vi "S4GUI.vi"() -> ()   [LabVIEW 2018] (continued)
            n2475 = call "Read WPROT.vi"("error in (no error)"=w5896, "Instrument in"=w5899) -> ("error out"=w5895:errorcluster, "Opt_Selector.lvclass"=w5897:refnum<class "Opt_Selector.lvclass">, "Instrument out"=w5898:refnum<class "Instrument.lvclass">)  [unwired: 7 in]
            n2476 = call-dynamic "Read sequencia_ant.vi"("error in (no error)"=w5895, "Opt_Selector in"=w5897) -> ("error out"=w5891:errorcluster, "sequencia_ant"=w5890:u16, "Opt_Selector out"=w5892:refnum<class "Opt_Selector.lvclass">)  [unwired: 7 in]
            n2477 = call-dynamic "Write sequencia.vi"("error in (no error)"=w5891, "sequencia"=w5890, "Opt_Selector in"=w5892) -> ("error out"=w5878:errorcluster, "Opt_Selector out"=w5881:refnum<class "Opt_Selector.lvclass">)  [unwired: 7 in]
            n2478 = call-dynamic "Read State Machine.vi"("error in (no error)"=w5878, "Device in"=w5881) -> ("error out"=w5883:errorcluster, "State Machine.lvclass"=w5886:refnum<class "State Machine.lvclass">, "Device out"=w5880:refnum<class "Opt_Selector.lvclass">)  [unwired: 7 in]
            n2479 = call "Next State.vi"("error in (no error)"=w5883, "New_State"=10, "State Machine in"=w5886) -> ("error out"=w5882:errorcluster, "State Machine out"=w5885:refnum<class "State Machine.lvclass">)  [unwired: 7 in]
            n2480 = call-dynamic "Write State Machine.vi"("error in (no error)"=w5882, "State Machine.lvclass"=w5885, "Device in"=w5880) -> ("error out"=w5877:errorcluster, "Device out"=w5879:refnum<class "Opt_Selector.lvclass">)  [unwired: 7 in]
            n2481 = call "Write WPROT.vi"("error in (no error)"=w5877, "Opt_Selector.lvclass"=w5879, "Instrument in"=w5898) -> ("error out"=w5894:errorcluster, "Instrument out"=w5893:refnum<class "Instrument.lvclass">)  [unwired: 7 in]
            n2482 = call "Write Instrument.lvclass.vi"("error in (no error)"=w5894, "Instrument.lvclass"=w5893, "S4ACS_GUI in"=w5900) -> ("error out"=w5888:errorcluster, "S4ACS_GUI out"=w5876:refnum<class "S4GUI.lvclass">)  [unwired: 7 in]
          }
          frame Enabled {
            w5931 = FALSE ("Wait Until Done")
            n2483 = call <vilib>:"Application Directory.vi"() -> ("Application Directory"=w5934:path)
            n2484 = Build Path(base path=w5934, name or relative path="MsgStop1.vi") -> (appended path=w5935:path)
            n2485 = Open VI Reference(vi path=w5935, error in (no error)=w5929) -> (vi reference=w5933:refnum<vi>, error out=w5932:errorcluster)  [unwired: 4 in]
            n2486 = invoke class="VI" method="Run VI"(reference=w5933, error in=w5932, "Wait until done"=w5931, "Auto Dispose Ref"=w5931) -> (error out=w5928:errorcluster)  [unwired: 1 in, 4 out]
          }
        }
      }
      event "Stop ch2": Value Change {
        n2487 = event-data() -> ()  [unwired: 1 in, 6 out]
        n2488 = disable-structure shown="Enabled" {
          disable-tunnel: w5940 -> [w5973 w5993]
          disable-tunnel: w5939 -> [w5971 w5995]
          disable-tunnel: [w5953 w5994] -> w5938
          disable-tunnel: [w5941 w5993] -> w5937
          frame Disabled {
            # "Para movimento \nda lamina retardadora"
            # "Restaura a última sequência de lâminas"
            n2489 = call "Read AcquisitionB.vi"("error in (no error)"=w5971, "S4ACS_GUI in"=w5973) -> ("error out"=w5975:errorcluster, "Acquisition.lvclass"=w5974:refnum<class "Acquisition.lvclass">, "S4ACS_GUI out"=w5972:refnum<class "S4GUI.lvclass">)  [unwired: 7 in]
            n2490 = disable-structure shown="Enabled" {
              disable-tunnel: w5975 -> [w5980 w5991]
              disable-tunnel: w5974 -> [w5979 w5992]
              disable-tunnel: [w5977 w5992] -> w5969
              disable-tunnel: [w5976 w5991] -> w5968
              frame Disabled {
                # "Só precisa enviar comando STOP quando\no controle dos ciclos for feito pelo ACS."
                n2491 = call-dynamic "Read Channel.vi"("error in (no error)"=w5980, "Acquisition in"=w5979) -> ("error out"=w5982:errorcluster, "Channel.lvclass"=w5981:refnum<class "Channel.lvclass">, "Acquisition out"=w5988:refnum<class "Acquisition.lvclass">)  [unwired: 7 in]
                n2492 = call-dynamic "Read State Machine.vi"("error in (no error)"=w5982, "Device in"=w5981) -> ("error out"=w5984:errorcluster, "State Machine.lvclass"=w5983:refnum<class "State Machine.lvclass">, "Device out"=w5986:refnum<class "Channel.lvclass">)  [unwired: 7 in]
                n2493 = call "Next State.vi"("error in (no error)"=w5984, "New_State"=u32 70, "State Machine in"=w5983) -> ("error out"=w5987:errorcluster, "State Machine out"=w5985:refnum<class "State Machine.lvclass">)  [unwired: 7 in]
                n2494 = call-dynamic "Write State Machine.vi"("error in (no error)"=w5987, "State Machine.lvclass"=w5985, "Device in"=w5986) -> ("error out"=w5989:errorcluster, "Device out"=w5990:refnum<class "Channel.lvclass">)  [unwired: 7 in]
                n2495 = call-dynamic "Write Channel.vi"("error in (no error)"=w5989, "Channel.lvclass"=w5990, "Acquisition in"=w5988) -> ("error out"=w5976:errorcluster, "Acquisition out"=w5977:refnum<class "Acquisition.lvclass">)  [unwired: 7 in]
              }
              frame Enabled {
                # "Não precisa enviar comando STOP para o ACS\nenquanto o controle dos ciclos for feito pela GUI."
              }
            }
            n2496 = call-dynamic "Write Acq_state.vi"("error in (no error)"=w5968, "Acq_state"=u32 0, "Acquisition in"=w5969) -> ("error out"=w5967:errorcluster, "Acquisition out"=w5966:refnum<class "Acquisition.lvclass">)  [unwired: 7 in]
            n2497 = call "Write AcquisitionB.vi"("error in (no error)"=w5967, "Acquisition.lvclass"=w5966, "S4ACS_GUI in"=w5972) -> ("error out"=w5954:errorcluster, "S4ACS_GUI out"=w5952:refnum<class "S4GUI.lvclass">)  [unwired: 7 in]
            n2498 = call "Read Instrument.lvclass.vi"("error in (no error)"=w5954, "S4ACS_GUI in"=w5952) -> ("error out"=w5961:errorcluster, "Instrument.lvclass"=w5964:refnum<class "Instrument.lvclass">, "S4ACS_GUI out"=w5965:refnum<class "S4GUI.lvclass">)  [unwired: 7 in]
            n2499 = call "Read WPROT.vi"("error in (no error)"=w5961, "Instrument in"=w5964) -> ("error out"=w5960:errorcluster, "Opt_Selector.lvclass"=w5962:refnum<class "Opt_Selector.lvclass">, "Instrument out"=w5963:refnum<class "Instrument.lvclass">)  [unwired: 7 in]
            n2500 = call-dynamic "Read sequencia_ant.vi"("error in (no error)"=w5960, "Opt_Selector in"=w5962) -> ("error out"=w5956:errorcluster, "sequencia_ant"=w5955:u16, "Opt_Selector out"=w5957:refnum<class "Opt_Selector.lvclass">)  [unwired: 7 in]
            n2501 = call-dynamic "Write sequencia.vi"("error in (no error)"=w5956, "sequencia"=w5955, "Opt_Selector in"=w5957) -> ("error out"=w5943:errorcluster, "Opt_Selector out"=w5946:refnum<class "Opt_Selector.lvclass">)  [unwired: 7 in]
            n2502 = call-dynamic "Read State Machine.vi"("error in (no error)"=w5943, "Device in"=w5946) -> ("error out"=w5948:errorcluster, "State Machine.lvclass"=w5951:refnum<class "State Machine.lvclass">, "Device out"=w5945:refnum<class "Opt_Selector.lvclass">)  [unwired: 7 in]
            n2503 = call "Next State.vi"("error in (no error)"=w5948, "New_State"=10, "State Machine in"=w5951) -> ("error out"=w5947:errorcluster, "State Machine out"=w5950:refnum<class "State Machine.lvclass">)  [unwired: 7 in]
            n2504 = call-dynamic "Write State Machine.vi"("error in (no error)"=w5947, "State Machine.lvclass"=w5950, "Device in"=w5945) -> ("error out"=w5942:errorcluster, "Device out"=w5944:refnum<class "Opt_Selector.lvclass">)  [unwired: 7 in]
            n2505 = call "Write WPROT.vi"("error in (no error)"=w5942, "Opt_Selector.lvclass"=w5944, "Instrument in"=w5963) -> ("error out"=w5959:errorcluster, "Instrument out"=w5958:refnum<class "Instrument.lvclass">)  [unwired: 7 in]
            n2506 = call "Write Instrument.lvclass.vi"("error in (no error)"=w5959, "Instrument.lvclass"=w5958, "S4ACS_GUI in"=w5965) -> ("error out"=w5953:errorcluster, "S4ACS_GUI out"=w5941:refnum<class "S4GUI.lvclass">)  [unwired: 7 in]
          }
          frame Enabled {
            w5997 = FALSE ("Wait Until Done")
            n2507 = call <vilib>:"Application Directory.vi"() -> ("Application Directory"=w6000:path)
            n2508 = Build Path(base path=w6000, name or relative path="MsgStop2.vi") -> (appended path=w6001:path)
            n2509 = Open VI Reference(vi path=w6001, error in (no error)=w5995) -> (vi reference=w5999:refnum<vi>, error out=w5998:errorcluster)  [unwired: 4 in]
            n2510 = invoke class="VI" method="Run VI"(reference=w5999, error in=w5998, "Wait until done"=w5997, "Auto Dispose Ref"=w5997) -> (error out=w5994:errorcluster)  [unwired: 1 in, 4 out]
          }
        }
      }
      event "Stop ch3": Value Change {
        n2511 = event-data() -> ()  [unwired: 1 in, 6 out]
        n2512 = disable-structure shown="Enabled" {
          disable-tunnel: w6005 -> [w6038 w6058]
          disable-tunnel: w6004 -> [w6036 w6060]
          disable-tunnel: [w6018 w6059] -> w6003
          disable-tunnel: [w6006 w6058] -> w6002
          frame Disabled {
            # "Para movimento \nda lamina retardadora"
            # "Restaura a última sequência de lâminas"
            n2513 = call-dynamic "Read AcquisitionC.vi"("error in (no error)"=w6036, "S4ACS_GUI in"=w6038) -> ("error out"=w6040:errorcluster, "Acquisition.lvclass"=w6039:refnum<class "Acquisition.lvclass">, "S4ACS_GUI out"=w6037:refnum<class "S4GUI.lvclass">)  [unwired: 7 in]
            n2514 = disable-structure shown="Enabled" {
              disable-tunnel: w6040 -> [w6045 w6056]
              disable-tunnel: w6039 -> [w6044 w6057]
              disable-tunnel: [w6042 w6057] -> w6034
              disable-tunnel: [w6041 w6056] -> w6033
              frame Disabled {
                # "Só precisa enviar comando STOP quando\no controle dos ciclos for feito pelo ACS."
                n2515 = call-dynamic "Read Channel.vi"("error in (no error)"=w6045, "Acquisition in"=w6044) -> ("error out"=w6047:errorcluster, "Channel.lvclass"=w6046:refnum<class "Channel.lvclass">, "Acquisition out"=w6053:refnum<class "Acquisition.lvclass">)  [unwired: 7 in]
                n2516 = call-dynamic "Read State Machine.vi"("error in (no error)"=w6047, "Device in"=w6046) -> ("error out"=w6049:errorcluster, "State Machine.lvclass"=w6048:refnum<class "State Machine.lvclass">, "Device out"=w6051:refnum<class "Channel.lvclass">)  [unwired: 7 in]
                n2517 = call "Next State.vi"("error in (no error)"=w6049, "New_State"=u32 70, "State Machine in"=w6048) -> ("error out"=w6052:errorcluster, "State Machine out"=w6050:refnum<class "State Machine.lvclass">)  [unwired: 7 in]
                n2518 = call-dynamic "Write State Machine.vi"("error in (no error)"=w6052, "State Machine.lvclass"=w6050, "Device in"=w6051) -> ("error out"=w6054:errorcluster, "Device out"=w6055:refnum<class "Channel.lvclass">)  [unwired: 7 in]
                n2519 = call-dynamic "Write Channel.vi"("error in (no error)"=w6054, "Channel.lvclass"=w6055, "Acquisition in"=w6053) -> ("error out"=w6041:errorcluster, "Acquisition out"=w6042:refnum<class "Acquisition.lvclass">)  [unwired: 7 in]
              }
              frame Enabled {
                # "Não precisa enviar comando STOP para o ACS\nenquanto o controle dos ciclos for feito pela GUI."
              }
            }
            n2520 = call-dynamic "Write Acq_state.vi"("error in (no error)"=w6033, "Acq_state"=u32 0, "Acquisition in"=w6034) -> ("error out"=w6032:errorcluster, "Acquisition out"=w6031:refnum<class "Acquisition.lvclass">)  [unwired: 7 in]
            n2521 = call-dynamic "Write AcquisitionC.vi"("error in (no error)"=w6032, "Acquisition.lvclass"=w6031, "S4ACS_GUI in"=w6037) -> ("error out"=w6019:errorcluster, "S4ACS_GUI out"=w6017:refnum<class "S4GUI.lvclass">)  [unwired: 7 in]
            n2522 = call "Read Instrument.lvclass.vi"("error in (no error)"=w6019, "S4ACS_GUI in"=w6017) -> ("error out"=w6026:errorcluster, "Instrument.lvclass"=w6029:refnum<class "Instrument.lvclass">, "S4ACS_GUI out"=w6030:refnum<class "S4GUI.lvclass">)  [unwired: 7 in]
            n2523 = call "Read WPROT.vi"("error in (no error)"=w6026, "Instrument in"=w6029) -> ("error out"=w6025:errorcluster, "Opt_Selector.lvclass"=w6027:refnum<class "Opt_Selector.lvclass">, "Instrument out"=w6028:refnum<class "Instrument.lvclass">)  [unwired: 7 in]
            n2524 = call-dynamic "Read sequencia_ant.vi"("error in (no error)"=w6025, "Opt_Selector in"=w6027) -> ("error out"=w6021:errorcluster, "sequencia_ant"=w6020:u16, "Opt_Selector out"=w6022:refnum<class "Opt_Selector.lvclass">)  [unwired: 7 in]
            n2525 = call-dynamic "Write sequencia.vi"("error in (no error)"=w6021, "sequencia"=w6020, "Opt_Selector in"=w6022) -> ("error out"=w6008:errorcluster, "Opt_Selector out"=w6011:refnum<class "Opt_Selector.lvclass">)  [unwired: 7 in]
            n2526 = call-dynamic "Read State Machine.vi"("error in (no error)"=w6008, "Device in"=w6011) -> ("error out"=w6013:errorcluster, "State Machine.lvclass"=w6016:refnum<class "State Machine.lvclass">, "Device out"=w6010:refnum<class "Opt_Selector.lvclass">)  [unwired: 7 in]
            n2527 = call "Next State.vi"("error in (no error)"=w6013, "New_State"=10, "State Machine in"=w6016) -> ("error out"=w6012:errorcluster, "State Machine out"=w6015:refnum<class "State Machine.lvclass">)  [unwired: 7 in]
            n2528 = call-dynamic "Write State Machine.vi"("error in (no error)"=w6012, "State Machine.lvclass"=w6015, "Device in"=w6010) -> ("error out"=w6007:errorcluster, "Device out"=w6009:refnum<class "Opt_Selector.lvclass">)  [unwired: 7 in]
            n2529 = call "Write WPROT.vi"("error in (no error)"=w6007, "Opt_Selector.lvclass"=w6009, "Instrument in"=w6028) -> ("error out"=w6024:errorcluster, "Instrument out"=w6023:refnum<class "Instrument.lvclass">)  [unwired: 7 in]
            n2530 = call "Write Instrument.lvclass.vi"("error in (no error)"=w6024, "Instrument.lvclass"=w6023, "S4ACS_GUI in"=w6030) -> ("error out"=w6018:errorcluster, "S4ACS_GUI out"=w6006:refnum<class "S4GUI.lvclass">)  [unwired: 7 in]
          }
          frame Enabled {
            w6062 = FALSE ("Wait Until Done")
            n2531 = call <vilib>:"Application Directory.vi"() -> ("Application Directory"=w6065:path)
            n2532 = Build Path(base path=w6065, name or relative path="MsgStop3.vi") -> (appended path=w6066:path)
            n2533 = Open VI Reference(vi path=w6066, error in (no error)=w6060) -> (vi reference=w6064:refnum<vi>, error out=w6063:errorcluster)  [unwired: 4 in]
            n2534 = invoke class="VI" method="Run VI"(reference=w6064, error in=w6063, "Wait until done"=w6062, "Auto Dispose Ref"=w6062) -> (error out=w6059:errorcluster)  [unwired: 1 in, 4 out]
          }
        }
      }
      event "Stop ch4": Value Change {
        n2535 = event-data() -> ()  [unwired: 1 in, 6 out]
        n2536 = disable-structure shown="Enabled" {
          disable-tunnel: w6070 -> [w6103 w6123]
          disable-tunnel: w6069 -> [w6101 w6125]
          disable-tunnel: [w6083 w6124] -> w6068
          disable-tunnel: [w6071 w6123] -> w6067
          frame Disabled {
            # "Para movimento \nda lamina retardadora"
            # "Restaura a última sequência de lâminas"
            n2537 = call-dynamic "Read AcquisitionD.vi"("error in (no error)"=w6101, "S4ACS_GUI in"=w6103) -> ("error out"=w6105:errorcluster, "Acquisition.lvclass"=w6104:refnum<class "Acquisition.lvclass">, "S4ACS_GUI out"=w6102:refnum<class "S4GUI.lvclass">)  [unwired: 7 in]
            n2538 = disable-structure shown="Enabled" {
              disable-tunnel: w6105 -> [w6110 w6121]
              disable-tunnel: w6104 -> [w6109 w6122]
              disable-tunnel: [w6107 w6122] -> w6099
              disable-tunnel: [w6106 w6121] -> w6098
              frame Disabled {
                # "Só precisa enviar comando STOP quando\no controle dos ciclos for feito pelo ACS."
                n2539 = call-dynamic "Read Channel.vi"("error in (no error)"=w6110, "Acquisition in"=w6109) -> ("error out"=w6112:errorcluster, "Channel.lvclass"=w6111:refnum<class "Channel.lvclass">, "Acquisition out"=w6118:refnum<class "Acquisition.lvclass">)  [unwired: 7 in]
                n2540 = call-dynamic "Read State Machine.vi"("error in (no error)"=w6112, "Device in"=w6111) -> ("error out"=w6114:errorcluster, "State Machine.lvclass"=w6113:refnum<class "State Machine.lvclass">, "Device out"=w6116:refnum<class "Channel.lvclass">)  [unwired: 7 in]
                n2541 = call "Next State.vi"("error in (no error)"=w6114, "New_State"=u32 70, "State Machine in"=w6113) -> ("error out"=w6117:errorcluster, "State Machine out"=w6115:refnum<class "State Machine.lvclass">)  [unwired: 7 in]
                n2542 = call-dynamic "Write State Machine.vi"("error in (no error)"=w6117, "State Machine.lvclass"=w6115, "Device in"=w6116) -> ("error out"=w6119:errorcluster, "Device out"=w6120:refnum<class "Channel.lvclass">)  [unwired: 7 in]
                n2543 = call-dynamic "Write Channel.vi"("error in (no error)"=w6119, "Channel.lvclass"=w6120, "Acquisition in"=w6118) -> ("error out"=w6106:errorcluster, "Acquisition out"=w6107:refnum<class "Acquisition.lvclass">)  [unwired: 7 in]
              }
              frame Enabled {
                # "Não precisa enviar comando STOP para o ACS\nenquanto o controle dos ciclos for feito pela GUI."
              }
            }
            n2544 = call-dynamic "Write Acq_state.vi"("error in (no error)"=w6098, "Acq_state"=u32 0, "Acquisition in"=w6099) -> ("error out"=w6097:errorcluster, "Acquisition out"=w6096:refnum<class "Acquisition.lvclass">)  [unwired: 7 in]
            n2545 = call-dynamic "Write AcquisitionD.vi"("error in (no error)"=w6097, "Acquisition.lvclass"=w6096, "S4ACS_GUI in"=w6102) -> ("error out"=w6084:errorcluster, "S4ACS_GUI out"=w6082:refnum<class "S4GUI.lvclass">)  [unwired: 7 in]
            n2546 = call "Read Instrument.lvclass.vi"("error in (no error)"=w6084, "S4ACS_GUI in"=w6082) -> ("error out"=w6091:errorcluster, "Instrument.lvclass"=w6094:refnum<class "Instrument.lvclass">, "S4ACS_GUI out"=w6095:refnum<class "S4GUI.lvclass">)  [unwired: 7 in]
            n2547 = call "Read WPROT.vi"("error in (no error)"=w6091, "Instrument in"=w6094) -> ("error out"=w6090:errorcluster, "Opt_Selector.lvclass"=w6092:refnum<class "Opt_Selector.lvclass">, "Instrument out"=w6093:refnum<class "Instrument.lvclass">)  [unwired: 7 in]
            n2548 = call-dynamic "Read sequencia_ant.vi"("error in (no error)"=w6090, "Opt_Selector in"=w6092) -> ("error out"=w6086:errorcluster, "sequencia_ant"=w6085:u16, "Opt_Selector out"=w6087:refnum<class "Opt_Selector.lvclass">)  [unwired: 7 in]
            n2549 = call-dynamic "Write sequencia.vi"("error in (no error)"=w6086, "sequencia"=w6085, "Opt_Selector in"=w6087) -> ("error out"=w6073:errorcluster, "Opt_Selector out"=w6076:refnum<class "Opt_Selector.lvclass">)  [unwired: 7 in]
            n2550 = call-dynamic "Read State Machine.vi"("error in (no error)"=w6073, "Device in"=w6076) -> ("error out"=w6078:errorcluster, "State Machine.lvclass"=w6081:refnum<class "State Machine.lvclass">, "Device out"=w6075:refnum<class "Opt_Selector.lvclass">)  [unwired: 7 in]
            n2551 = call "Next State.vi"("error in (no error)"=w6078, "New_State"=10, "State Machine in"=w6081) -> ("error out"=w6077:errorcluster, "State Machine out"=w6080:refnum<class "State Machine.lvclass">)  [unwired: 7 in]
            n2552 = call-dynamic "Write State Machine.vi"("error in (no error)"=w6077, "State Machine.lvclass"=w6080, "Device in"=w6075) -> ("error out"=w6072:errorcluster, "Device out"=w6074:refnum<class "Opt_Selector.lvclass">)  [unwired: 7 in]
            n2553 = call "Write WPROT.vi"("error in (no error)"=w6072, "Opt_Selector.lvclass"=w6074, "Instrument in"=w6093) -> ("error out"=w6089:errorcluster, "Instrument out"=w6088:refnum<class "Instrument.lvclass">)  [unwired: 7 in]
            n2554 = call "Write Instrument.lvclass.vi"("error in (no error)"=w6089, "Instrument.lvclass"=w6088, "S4ACS_GUI in"=w6095) -> ("error out"=w6083:errorcluster, "S4ACS_GUI out"=w6071:refnum<class "S4GUI.lvclass">)  [unwired: 7 in]
          }
          frame Enabled {
            w6127 = FALSE ("Wait Until Done")
            n2555 = call <vilib>:"Application Directory.vi"() -> ("Application Directory"=w6130:path)
            n2556 = Build Path(base path=w6130, name or relative path="MsgStop4.vi") -> (appended path=w6131:path)
            n2557 = Open VI Reference(vi path=w6131, error in (no error)=w6125) -> (vi reference=w6129:refnum<vi>, error out=w6128:errorcluster)  [unwired: 4 in]
            n2558 = invoke class="VI" method="Run VI"(reference=w6129, error in=w6128, "Wait until done"=w6127, "Auto Dispose Ref"=w6127) -> (error out=w6124:errorcluster)  [unwired: 1 in, 4 out]
          }
        }
      }
      event "Pause ch1": Value Change {
        n2559 = event-data() -> ()  [unwired: 1 in, 6 out]
        n2560 = disable-structure shown="Enabled" {
          disable-tunnel: w6135 -> [w6151 w6162]
          disable-tunnel: [w6149 w6160] -> w6134
          disable-tunnel: w6133 -> [w6148 w6161]
          disable-tunnel: [w6136 w6162] -> w6132
          frame Disabled {
            n2561 = call-dynamic "Read AcquisitionA.vi"("error in (no error)"=w6148, "S4ACS_GUI in"=w6151) -> ("error out"=w6143:errorcluster, "Acquisition.lvclass"=w6142:refnum<class "Acquisition.lvclass">, "S4ACS_GUI out"=w6150:refnum<class "S4GUI.lvclass">)  [unwired: 7 in]
            n2562 = call-dynamic "Read Acq_state.vi"("error in (no error)"=w6143, "Acquisition in"=w6142) -> ("error out"=w6145:errorcluster, "Acq_state"=w6146:u32, "Acquisition out"=w6147:refnum<class "Acquisition.lvclass">)  [unwired: 7 in]
            n2563 = call-dynamic "Write Acq_prevstate.vi"("error in (no error)"=w6145, "Acq_prevstate"=w6146, "Acquisition in"=w6147) -> ("error out"=w6140:errorcluster, "Acquisition out"=w6141:refnum<class "Acquisition.lvclass">)  [unwired: 7 in]
            n2564 = call-dynamic "Write Acq_state.vi"("error in (no error)"=w6140, "Acq_state"=u32 400, "Acquisition in"=w6141) -> ("error out"=w6138:errorcluster, "Acquisition out"=w6139:refnum<class "Acquisition.lvclass">)  [unwired: 7 in]
            n2565 = disable-structure shown="Enabled" {
              disable-tunnel: w6138 -> [w6153 w6159]
              disable-tunnel: [w6152 w6159] -> w6137
              frame Disabled {
                n2566 = property on="Start ch1" class="Bool"(error in=w6153, "BoolText.Text"="RESUME" ("Caption.Text")) -> (error out=w6157:errorcluster)  [unwired: 1 in, 1 out]
                n2567 = property on="Pause ch1" class="Bool"(error in=w6157, "DisabledEnum"=T7."Disabled and Grayed Out" ("Disabled")) -> (error out=w6158:errorcluster)  [unwired: 1 in, 1 out]
                n2568 = property on="Start ch1" class="Bool"(error in=w6158, "DisabledEnum"=T7."Enabled" ("Disabled")) -> (error out=w6152:errorcluster)  [unwired: 1 in, 1 out]
              }
              frame Enabled {
              }
            }
            n2569 = call-dynamic "Write AcquisitionA.vi"("error in (no error)"=w6137, "Acquisition.lvclass"=w6139, "S4ACS_GUI in"=w6150) -> ("error out"=w6149:errorcluster, "S4ACS_GUI out"=w6136:refnum<class "S4GUI.lvclass">)  [unwired: 7 in]
          }
          frame Enabled {
            w6164 = FALSE ("Wait Until Done")
            n2570 = call <vilib>:"Application Directory.vi"() -> ("Application Directory"=w6167:path)
            n2571 = Build Path(base path=w6167, name or relative path="MsgPause1.vi") -> (appended path=w6168:path)
            n2572 = Open VI Reference(vi path=w6168, error in (no error)=w6161) -> (vi reference=w6166:refnum<vi>, error out=w6165:errorcluster)  [unwired: 4 in]
            n2573 = invoke class="VI" method="Run VI"(reference=w6166, error in=w6165, "Wait until done"=w6164, "Auto Dispose Ref"=w6164) -> (error out=w6160:errorcluster)  [unwired: 1 in, 4 out]
          }
        }
      }
      event "Pause ch2": Value Change {
        n2574 = event-data() -> ()  [unwired: 1 in, 6 out]
        n2575 = disable-structure shown="Enabled" {
          disable-tunnel: w6172 -> [w6187 w6188]
          disable-tunnel: [w6185 w6189] -> w6171
          disable-tunnel: w6170 -> [w6184 w6190]
          disable-tunnel: [w6174 w6188] -> w6169
          frame Disabled {
            n2576 = call "Read AcquisitionB.vi"("error in (no error)"=w6184, "S4ACS_GUI in"=w6187) -> ("error out"=w6179:errorcluster, "Acquisition.lvclass"=w6178:refnum<class "Acquisition.lvclass">, "S4ACS_GUI out"=w6186:refnum<class "S4GUI.lvclass">)  [unwired: 7 in]
            n2577 = call-dynamic "Read Acq_state.vi"("error in (no error)"=w6179, "Acquisition in"=w6178) -> ("error out"=w6181:errorcluster, "Acq_state"=w6182:u32, "Acquisition out"=w6183:refnum<class "Acquisition.lvclass">)  [unwired: 7 in]
            n2578 = call-dynamic "Write Acq_prevstate.vi"("error in (no error)"=w6181, "Acq_prevstate"=w6182, "Acquisition in"=w6183) -> ("error out"=w6176:errorcluster, "Acquisition out"=w6177:refnum<class "Acquisition.lvclass">)  [unwired: 7 in]
            n2579 = call-dynamic "Write Acq_state.vi"("error in (no error)"=w6176, "Acq_state"=u32 400, "Acquisition in"=w6177) -> ("error out"=w6173:errorcluster, "Acquisition out"=w6175:refnum<class "Acquisition.lvclass">)  [unwired: 7 in]
            n2580 = call "Write AcquisitionB.vi"("error in (no error)"=w6173, "Acquisition.lvclass"=w6175, "S4ACS_GUI in"=w6186) -> ("error out"=w6185:errorcluster, "S4ACS_GUI out"=w6174:refnum<class "S4GUI.lvclass">)  [unwired: 7 in]
          }
          frame Enabled {
            w6192 = FALSE ("Wait Until Done")
            n2581 = call <vilib>:"Application Directory.vi"() -> ("Application Directory"=w6195:path)
            n2582 = Build Path(base path=w6195, name or relative path="MsgPause2.vi") -> (appended path=w6196:path)
            n2583 = Open VI Reference(vi path=w6196, error in (no error)=w6190) -> (vi reference=w6194:refnum<vi>, error out=w6193:errorcluster)  [unwired: 4 in]
            n2584 = invoke class="VI" method="Run VI"(reference=w6194, error in=w6193, "Wait until done"=w6192, "Auto Dispose Ref"=w6192) -> (error out=w6189:errorcluster)  [unwired: 1 in, 4 out]
          }
        }
      }
      event "Pause ch3": Value Change {
        n2585 = event-data() -> ()  [unwired: 1 in, 6 out]
        n2586 = disable-structure shown="Enabled" {
          disable-tunnel: w6200 -> [w6215 w6216]
          disable-tunnel: [w6213 w6217] -> w6199
          disable-tunnel: w6198 -> [w6212 w6218]
          disable-tunnel: [w6202 w6216] -> w6197
          frame Disabled {
            n2587 = call-dynamic "Read AcquisitionC.vi"("error in (no error)"=w6212, "S4ACS_GUI in"=w6215) -> ("error out"=w6207:errorcluster, "Acquisition.lvclass"=w6206:refnum<class "Acquisition.lvclass">, "S4ACS_GUI out"=w6214:refnum<class "S4GUI.lvclass">)  [unwired: 7 in]
            n2588 = call-dynamic "Read Acq_state.vi"("error in (no error)"=w6207, "Acquisition in"=w6206) -> ("error out"=w6209:errorcluster, "Acq_state"=w6210:u32, "Acquisition out"=w6211:refnum<class "Acquisition.lvclass">)  [unwired: 7 in]
            n2589 = call-dynamic "Write Acq_prevstate.vi"("error in (no error)"=w6209, "Acq_prevstate"=w6210, "Acquisition in"=w6211) -> ("error out"=w6204:errorcluster, "Acquisition out"=w6205:refnum<class "Acquisition.lvclass">)  [unwired: 7 in]
            n2590 = call-dynamic "Write Acq_state.vi"("error in (no error)"=w6204, "Acq_state"=u32 400, "Acquisition in"=w6205) -> ("error out"=w6201:errorcluster, "Acquisition out"=w6203:refnum<class "Acquisition.lvclass">)  [unwired: 7 in]
            n2591 = call-dynamic "Write AcquisitionC.vi"("error in (no error)"=w6201, "Acquisition.lvclass"=w6203, "S4ACS_GUI in"=w6214) -> ("error out"=w6213:errorcluster, "S4ACS_GUI out"=w6202:refnum<class "S4GUI.lvclass">)  [unwired: 7 in]
          }
          frame Enabled {
            w6220 = FALSE ("Wait Until Done")
            n2592 = call <vilib>:"Application Directory.vi"() -> ("Application Directory"=w6223:path)
            n2593 = Build Path(base path=w6223, name or relative path="MsgPause3.vi") -> (appended path=w6224:path)
            n2594 = Open VI Reference(vi path=w6224, error in (no error)=w6218) -> (vi reference=w6222:refnum<vi>, error out=w6221:errorcluster)  [unwired: 4 in]
            n2595 = invoke class="VI" method="Run VI"(reference=w6222, error in=w6221, "Wait until done"=w6220, "Auto Dispose Ref"=w6220) -> (error out=w6217:errorcluster)  [unwired: 1 in, 4 out]
          }
        }
      }
      event "Pause ch4": Value Change {
        n2596 = event-data() -> ()  [unwired: 1 in, 6 out]
        n2597 = disable-structure shown="Enabled" {
          disable-tunnel: w6228 -> [w6243 w6252]
          disable-tunnel: [w6241 w6244] -> w6227
          disable-tunnel: w6226 -> [w6240 w6245]
          disable-tunnel: [w6230 w6252] -> w6225
          frame Disabled {
            n2598 = call-dynamic "Read AcquisitionD.vi"("error in (no error)"=w6240, "S4ACS_GUI in"=w6243) -> ("error out"=w6235:errorcluster, "Acquisition.lvclass"=w6234:refnum<class "Acquisition.lvclass">, "S4ACS_GUI out"=w6242:refnum<class "S4GUI.lvclass">)  [unwired: 7 in]
            n2599 = call-dynamic "Read Acq_state.vi"("error in (no error)"=w6235, "Acquisition in"=w6234) -> ("error out"=w6237:errorcluster, "Acq_state"=w6238:u32, "Acquisition out"=w6239:refnum<class "Acquisition.lvclass">)  [unwired: 7 in]
            n2600 = call-dynamic "Write Acq_prevstate.vi"("error in (no error)"=w6237, "Acq_prevstate"=w6238, "Acquisition in"=w6239) -> ("error out"=w6232:errorcluster, "Acquisition out"=w6233:refnum<class "Acquisition.lvclass">)  [unwired: 7 in]
            n2601 = call-dynamic "Write Acq_state.vi"("error in (no error)"=w6232, "Acq_state"=u32 400, "Acquisition in"=w6233) -> ("error out"=w6229:errorcluster, "Acquisition out"=w6231:refnum<class "Acquisition.lvclass">)  [unwired: 7 in]
            n2602 = call-dynamic "Write AcquisitionD.vi"("error in (no error)"=w6229, "Acquisition.lvclass"=w6231, "S4ACS_GUI in"=w6242) -> ("error out"=w6241:errorcluster, "S4ACS_GUI out"=w6230:refnum<class "S4GUI.lvclass">)  [unwired: 7 in]
          }
          frame Enabled {
            w6247 = FALSE ("Wait Until Done")
            n2603 = call <vilib>:"Application Directory.vi"() -> ("Application Directory"=w6250:path)
            n2604 = Build Path(base path=w6250, name or relative path="MsgPause4.vi") -> (appended path=w6251:path)
            n2605 = Open VI Reference(vi path=w6251, error in (no error)=w6245) -> (vi reference=w6249:refnum<vi>, error out=w6248:errorcluster)  [unwired: 4 in]
            n2606 = invoke class="VI" method="Run VI"(reference=w6249, error in=w6248, "Wait until done"=w6247, "Auto Dispose Ref"=w6247) -> (error out=w6244:errorcluster)  [unwired: 1 in, 4 out]
          }
        }
      }
      event "Stop SM": Value Change {
        w6253 = 0.0 ("Scale.Range:Minor Increment")
        n2607 = event-data() -> ()  [unwired: 1 in, 6 out]
        n2608 = disable-structure shown="Enabled" {
          disable-tunnel: w6258 -> [w6292 w6315]
          disable-tunnel: w6257 -> [w6290 w6316]
          disable-tunnel: [w6277 w6314] -> w6255
          disable-tunnel: [w6261 w6315] -> w6254
          frame Disabled {
            # "Não precisa enviar comando STOP para o ACS\nenquanto o controle dos ciclos for feito pela GUI."
            # "Para movimento \nda lamina retardadora"
            # "Restaura a sequencia anterior"
            n2609 = call-dynamic "Read AcquisitionA.vi"("error in (no error)"=w6290, "S4ACS_GUI in"=w6292) -> ("error out"=w6294:errorcluster, "Acquisition.lvclass"=w6293:refnum<class "Acquisition.lvclass">, "S4ACS_GUI out"=w6291:refnum<class "S4GUI.lvclass">)  [unwired: 7 in]
            n2610 = disable-structure shown="Enabled" {
              disable-tunnel: [w6308 w6312] -> w6296
              disable-tunnel: [w6307 w6313] -> w6295
              disable-tunnel: w6294 -> [w6299 w6312]
              disable-tunnel: w6293 -> [w6298 w6313]
              frame Disabled {
                n2611 = call-dynamic "Read Channel.vi"("error in (no error)"=w6299, "Acquisition in"=w6298) -> ("error out"=w6301:errorcluster, "Channel.lvclass"=w6300:refnum<class "Channel.lvclass">, "Acquisition out"=w6309:refnum<class "Acquisition.lvclass">)  [unwired: 7 in]
                n2612 = call-dynamic "Read State Machine.vi"("error in (no error)"=w6301, "Device in"=w6300) -> ("error out"=w6303:errorcluster, "State Machine.lvclass"=w6302:refnum<class "State Machine.lvclass">, "Device out"=w6305:refnum<class "Channel.lvclass">)  [unwired: 7 in]
                n2613 = call "Next State.vi"("error in (no error)"=w6303, "New_State"=u32 70, "State Machine in"=w6302) -> ("error out"=w6306:errorcluster, "State Machine out"=w6304:refnum<class "State Machine.lvclass">)  [unwired: 7 in]
                n2614 = call-dynamic "Write State Machine.vi"("error in (no error)"=w6306, "State Machine.lvclass"=w6304, "Device in"=w6305) -> ("error out"=w6310:errorcluster, "Device out"=w6311:refnum<class "Channel.lvclass">)  [unwired: 7 in]
                n2615 = call-dynamic "Write Channel.vi"("error in (no error)"=w6310, "Channel.lvclass"=w6311, "Acquisition in"=w6309) -> ("error out"=w6308:errorcluster, "Acquisition out"=w6307:refnum<class "Acquisition.lvclass">)  [unwired: 7 in]
              }
              frame Enabled {
              }
            }
            n2616 = call-dynamic "Write AcquisitionA.vi"("error in (no error)"=w6296, "Acquisition.lvclass"=w6295, "S4ACS_GUI in"=w6291) -> ("error out"=w6259:errorcluster, "S4ACS_GUI out"=w6260:refnum<class "S4GUI.lvclass">)  [unwired: 7 in]
            n2617 = call-dynamic "Write Obs_state.vi"("error in (no error)"=w6259, "Obs_state"=u32 0, "S4ACS_GUI in"=w6260) -> ("error out"=w6279:errorcluster, "S4ACS_GUI out"=w6280:refnum<class "S4GUI.lvclass">)  [unwired: 7 in]
            n2618 = call "Read Instrument.lvclass.vi"("error in (no error)"=w6279, "S4ACS_GUI in"=w6280) -> ("error out"=w6288:errorcluster, "Instrument.lvclass"=w6286:refnum<class "Instrument.lvclass">, "S4ACS_GUI out"=w6287:refnum<class "S4GUI.lvclass">)  [unwired: 7 in]
            n2619 = call "Read WPROT.vi"("error in (no error)"=w6288, "Instrument in"=w6286) -> ("error out"=w6273:errorcluster, "Opt_Selector.lvclass"=w6276:refnum<class "Opt_Selector.lvclass">, "Instrument out"=w6285:refnum<class "Instrument.lvclass">)  [unwired: 7 in]
            n2620 = call-dynamic "Read sequencia_ant.vi"("error in (no error)"=w6273, "Opt_Selector in"=w6276) -> ("error out"=w6272:errorcluster, "sequencia_ant"=w6274:u16, "Opt_Selector out"=w6275:refnum<class "Opt_Selector.lvclass">)  [unwired: 7 in]
            n2621 = call-dynamic "Write sequencia.vi"("error in (no error)"=w6272, "sequencia"=w6274, "Opt_Selector in"=w6275) -> ("error out"=w6270:errorcluster, "Opt_Selector out"=w6271:refnum<class "Opt_Selector.lvclass">)  [unwired: 7 in]
            n2622 = call-dynamic "Read State Machine.vi"("error in (no error)"=w6270, "Device in"=w6271) -> ("error out"=w6265:errorcluster, "State Machine.lvclass"=w6268:refnum<class "State Machine.lvclass">, "Device out"=w6269:refnum<class "Opt_Selector.lvclass">)  [unwired: 7 in]
            n2623 = call "Next State.vi"("error in (no error)"=w6265, "New_State"=10, "State Machine in"=w6268) -> ("error out"=w6264:errorcluster, "State Machine out"=w6267:refnum<class "State Machine.lvclass">)  [unwired: 7 in]
            n2624 = call-dynamic "Write State Machine.vi"("error in (no error)"=w6264, "State Machine.lvclass"=w6267, "Device in"=w6269) -> ("error out"=w6263:errorcluster, "Device out"=w6262:refnum<class "Opt_Selector.lvclass">)  [unwired: 7 in]
            n2625 = call "Write WPROT.vi"("error in (no error)"=w6263, "Opt_Selector.lvclass"=w6262, "Instrument in"=w6285) -> ("error out"=w6283:errorcluster, "Instrument out"=w6284:refnum<class "Instrument.lvclass">)  [unwired: 7 in]
            n2626 = call "Write Instrument.lvclass.vi"("error in (no error)"=w6283, "Instrument.lvclass"=w6284, "S4ACS_GUI in"=w6287) -> ("error out"=w6282:errorcluster, "S4ACS_GUI out"=w6281:refnum<class "S4GUI.lvclass">)  [unwired: 7 in]
            n2627 = call-dynamic "Write ciclos.vi"("error in (no error)"=w6282, "ciclos"=u32 0, "S4ACS_GUI in"=w6281) -> ("error out"=w6277:errorcluster, "S4ACS_GUI out"=w6261:refnum<class "S4GUI.lvclass">)  [unwired: 7 in]
          }
          frame Enabled {
            w6318 = FALSE ("Wait Until Done")
            n2628 = call <vilib>:"Application Directory.vi"() -> ("Application Directory"=w6321:path)
            n2629 = Build Path(base path=w6321, name or relative path="MsgStopSync.vi") -> (appended path=w6322:path)
            n2630 = Open VI Reference(vi path=w6322, error in (no error)=w6316) -> (vi reference=w6320:refnum<vi>, error out=w6319:errorcluster)  [unwired: 4 in]
            n2631 = invoke class="VI" method="Run VI"(reference=w6320, error in=w6319, "Wait until done"=w6318, "Auto Dispose Ref"=w6318) -> (error out=w6314:errorcluster)  [unwired: 1 in, 4 out]
          }
        }
        n2632 = property on="#Cycles Done" class="Slide (strict)"(error in=w6255, "Scale.Maximum"=w6253, "Scale.Minimum"=w6253) -> (error out=w6256:errorcluster)  [unwired: 1 in, 1 out]
      }
      event "Abort SM": Value Change {
        w6325 = 0.0 ("Scale.Range:Minor Increment")
        n2633 = event-data() -> ()  [unwired: 1 in, 6 out]
        n2634 = disable-structure shown="Enabled" {
          disable-tunnel: w6328 -> [w6418 w6441]
          disable-tunnel: w6327 -> [w6416 w6443]
          disable-tunnel: [w6330 w6441] -> w6324
          disable-tunnel: [w6329 w6442] -> w6323
          frame Disabled {
            # "Restaura a sequencia anterior"
            # "Para movimento \nda lamina retardadora"
            n2635 = call-dynamic "Read AcquisitionA.vi"("error in (no error)"=w6416, "S4ACS_GUI in"=w6418) -> ("error out"=w6421:errorcluster, "Acquisition.lvclass"=w6420:refnum<class "Acquisition.lvclass">, "S4ACS_GUI out"=w6417:refnum<class "S4GUI.lvclass">)  [unwired: 7 in]
            n2636 = call-dynamic "Read Channel.vi"("error in (no error)"=w6421, "Acquisition in"=w6420) -> ("error out"=w6423:errorcluster, "Channel.lvclass"=w6422:refnum<class "Channel.lvclass">, "Acquisition out"=w6431:refnum<class "Acquisition.lvclass">)  [unwired: 7 in]
            n2637 = call-dynamic "Read State Machine.vi"("error in (no error)"=w6423, "Device in"=w6422) -> ("error out"=w6425:errorcluster, "State Machine.lvclass"=w6424:refnum<class "State Machine.lvclass">, "Device out"=w6427:refnum<class "Channel.lvclass">)  [unwired: 7 in]
            n2638 = call "Next State.vi"("error in (no error)"=w6425, "New_State"=u32 80, "State Machine in"=w6424) -> ("error out"=w6428:errorcluster, "State Machine out"=w6426:refnum<class "State Machine.lvclass">)  [unwired: 7 in]
            n2639 = call-dynamic "Write State Machine.vi"("error in (no error)"=w6428, "State Machine.lvclass"=w6426, "Device in"=w6427) -> ("error out"=w6432:errorcluster, "Device out"=w6433:refnum<class "Channel.lvclass">)  [unwired: 7 in]
            n2640 = call-dynamic "Write Channel.vi"("error in (no error)"=w6432, "Channel.lvclass"=w6433, "Acquisition in"=w6431) -> ("error out"=w6430:errorcluster, "Acquisition out"=w6429:refnum<class "Acquisition.lvclass">)  [unwired: 7 in]
            n2641 = call-dynamic "Write AcquisitionA.vi"("error in (no error)"=w6430, "Acquisition.lvclass"=w6429, "S4ACS_GUI in"=w6417) -> ("error out"=w6402:errorcluster, "S4ACS_GUI out"=w6401:refnum<class "S4GUI.lvclass">)  [unwired: 7 in]
            n2642 = call "Read AcquisitionB.vi"("error in (no error)"=w6402, "S4ACS_GUI in"=w6401) -> ("error out"=w6395:errorcluster, "Acquisition.lvclass"=w6399:refnum<class "Acquisition.lvclass">, "S4ACS_GUI out"=w6400:refnum<class "S4GUI.lvclass">)  [unwired: 7 in]
            n2643 = call-dynamic "Read Channel.vi"("error in (no error)"=w6395, "Acquisition in"=w6399) -> ("error out"=w6410:errorcluster, "Channel.lvclass"=w6411:refnum<class "Channel.lvclass">, "Acquisition out"=w6397:refnum<class "Acquisition.lvclass">)  [unwired: 7 in]
            n2644 = call-dynamic "Read State Machine.vi"("error in (no error)"=w6410, "Device in"=w6411) -> ("error out"=w6408:errorcluster, "State Machine.lvclass"=w6409:refnum<class "State Machine.lvclass">, "Device out"=w6406:refnum<class "Channel.lvclass">)  [unwired: 7 in]
            n2645 = call "Next State.vi"("error in (no error)"=w6408, "New_State"=u32 80, "State Machine in"=w6409) -> ("error out"=w6405:errorcluster, "State Machine out"=w6407:refnum<class "State Machine.lvclass">)  [unwired: 7 in]
            n2646 = call-dynamic "Write State Machine.vi"("error in (no error)"=w6405, "State Machine.lvclass"=w6407, "Device in"=w6406) -> ("error out"=w6404:errorcluster, "Device out"=w6403:refnum<class "Channel.lvclass">)  [unwired: 7 in]
            n2647 = call-dynamic "Write Channel.vi"("error in (no error)"=w6404, "Channel.lvclass"=w6403, "Acquisition in"=w6397) -> ("error out"=w6396:errorcluster, "Acquisition out"=w6398:refnum<class "Acquisition.lvclass">)  [unwired: 7 in]
            n2648 = call "Write AcquisitionB.vi"("error in (no error)"=w6396, "Acquisition.lvclass"=w6398, "S4ACS_GUI in"=w6400) -> ("error out"=w6362:errorcluster, "S4ACS_GUI out"=w6361:refnum<class "S4GUI.lvclass">)  [unwired: 7 in]
            n2649 = call-dynamic "Read AcquisitionC.vi"("error in (no error)"=w6362, "S4ACS_GUI in"=w6361) -> ("error out"=w6379:errorcluster, "Acquisition.lvclass"=w6383:refnum<class "Acquisition.lvclass">, "S4ACS_GUI out"=w6384:refnum<class "S4GUI.lvclass">)  [unwired: 7 in]
            n2650 = call-dynamic "Read Channel.vi"("error in (no error)"=w6379, "Acquisition in"=w6383) -> ("error out"=w6392:errorcluster, "Channel.lvclass"=w6393:refnum<class "Channel.lvclass">, "Acquisition out"=w6381:refnum<class "Acquisition.lvclass">)  [unwired: 7 in]
            n2651 = call-dynamic "Read State Machine.vi"("error in (no error)"=w6392, "Device in"=w6393) -> ("error out"=w6390:errorcluster, "State Machine.lvclass"=w6391:refnum<class "State Machine.lvclass">, "Device out"=w6388:refnum<class "Channel.lvclass">)  [unwired: 7 in]
            n2652 = call "Next State.vi"("error in (no error)"=w6390, "New_State"=u32 80, "State Machine in"=w6391) -> ("error out"=w6387:errorcluster, "State Machine out"=w6389:refnum<class "State Machine.lvclass">)  [unwired: 7 in]
            n2653 = call-dynamic "Write State Machine.vi"("error in (no error)"=w6387, "State Machine.lvclass"=w6389, "Device in"=w6388) -> ("error out"=w6386:errorcluster, "Device out"=w6385:refnum<class "Channel.lvclass">)  [unwired: 7 in]
            n2654 = call-dynamic "Write Channel.vi"("error in (no error)"=w6386, "Channel.lvclass"=w6385, "Acquisition in"=w6381) -> ("error out"=w6380:errorcluster, "Acquisition out"=w6382:refnum<class "Acquisition.lvclass">)  [unwired: 7 in]
            n2655 = call-dynamic "Write AcquisitionC.vi"("error in (no error)"=w6380, "Acquisition.lvclass"=w6382, "S4ACS_GUI in"=w6384) -> ("error out"=w6360:errorcluster, "S4ACS_GUI out"=w6359:refnum<class "S4GUI.lvclass">)  [unwired: 7 in]
            n2656 = call-dynamic "Read AcquisitionD.vi"("error in (no error)"=w6360, "S4ACS_GUI in"=w6359) -> ("error out"=w6363:errorcluster, "Acquisition.lvclass"=w6367:refnum<class "Acquisition.lvclass">, "S4ACS_GUI out"=w6368:refnum<class "S4GUI.lvclass">)  [unwired: 7 in]
            n2657 = call-dynamic "Read Channel.vi"("error in (no error)"=w6363, "Acquisition in"=w6367) -> ("error out"=w6376:errorcluster, "Channel.lvclass"=w6377:refnum<class "Channel.lvclass">, "Acquisition out"=w6365:refnum<class "Acquisition.lvclass">)  [unwired: 7 in]
            n2658 = call-dynamic "Read State Machine.vi"("error in (no error)"=w6376, "Device in"=w6377) -> ("error out"=w6374:errorcluster, "State Machine.lvclass"=w6375:refnum<class "State Machine.lvclass">, "Device out"=w6372:refnum<class "Channel.lvclass">)  [unwired: 7 in]
            n2659 = call "Next State.vi"("error in (no error)"=w6374, "New_State"=u32 80, "State Machine in"=w6375) -> ("error out"=w6371:errorcluster, "State Machine out"=w6373:refnum<class "State Machine.lvclass">)  [unwired: 7 in]
            n2660 = call-dynamic "Write State Machine.vi"("error in (no error)"=w6371, "State Machine.lvclass"=w6373, "Device in"=w6372) -> ("error out"=w6370:errorcluster, "Device out"=w6369:refnum<class "Channel.lvclass">)  [unwired: 7 in]
            n2661 = call-dynamic "Write Channel.vi"("error in (no error)"=w6370, "Channel.lvclass"=w6369, "Acquisition in"=w6365) -> ("error out"=w6364:errorcluster, "Acquisition out"=w6366:refnum<class "Acquisition.lvclass">)  [unwired: 7 in]
            n2662 = call-dynamic "Write AcquisitionD.vi"("error in (no error)"=w6364, "Acquisition.lvclass"=w6366, "S4ACS_GUI in"=w6368) -> ("error out"=w6357:errorcluster, "S4ACS_GUI out"=w6358:refnum<class "S4GUI.lvclass">)  [unwired: 7 in]
            n2663 = disable-structure shown="Enabled" {
              disable-tunnel: w6358 -> [w6438 w6440]
              disable-tunnel: w6357 -> [w6437 w6439]
              disable-tunnel: [w6435 w6440] -> w6414
              disable-tunnel: [w6434 w6439] -> w6413
              frame Disabled {
                n2664 = call-dynamic "Write aborted.vi"("error in (no error)"=w6437, "aborted"=TRUE ("stopped"), "S4ACS_GUI in"=w6438) -> ("error out"=w6434:errorcluster, "S4ACS_GUI out"=w6435:refnum<class "S4GUI.lvclass">)  [unwired: 7 in]
              }
              frame Enabled {
              }
            }
            n2665 = call-dynamic "Write Obs_state.vi"("error in (no error)"=w6413, "Obs_state"=u32 0, "S4ACS_GUI in"=w6414) -> ("error out"=w6331:errorcluster, "S4ACS_GUI out"=w6332:refnum<class "S4GUI.lvclass">)  [unwired: 7 in]
            n2666 = call "Read Instrument.lvclass.vi"("error in (no error)"=w6331, "S4ACS_GUI in"=w6332) -> ("error out"=w6351:errorcluster, "Instrument.lvclass"=w6353:refnum<class "Instrument.lvclass">, "S4ACS_GUI out"=w6352:refnum<class "S4GUI.lvclass">)  [unwired: 7 in]
            n2667 = call "Read WPROT.vi"("error in (no error)"=w6351, "Instrument in"=w6353) -> ("error out"=w6346:errorcluster, "Opt_Selector.lvclass"=w6349:refnum<class "Opt_Selector.lvclass">, "Instrument out"=w6354:refnum<class "Instrument.lvclass">)  [unwired: 7 in]
            n2668 = call-dynamic "Read sequencia_ant.vi"("error in (no error)"=w6346, "Opt_Selector in"=w6349) -> ("error out"=w6345:errorcluster, "sequencia_ant"=w6347:u16, "Opt_Selector out"=w6348:refnum<class "Opt_Selector.lvclass">)  [unwired: 7 in]
            n2669 = call-dynamic "Write sequencia.vi"("error in (no error)"=w6345, "sequencia"=w6347, "Opt_Selector in"=w6348) -> ("error out"=w6340:errorcluster, "Opt_Selector out"=w6341:refnum<class "Opt_Selector.lvclass">)  [unwired: 7 in]
            n2670 = call-dynamic "Read State Machine.vi"("error in (no error)"=w6340, "Device in"=w6341) -> ("error out"=w6343:errorcluster, "State Machine.lvclass"=w6338:refnum<class "State Machine.lvclass">, "Device out"=w6339:refnum<class "Opt_Selector.lvclass">)  [unwired: 7 in]
            n2671 = call "Next State.vi"("error in (no error)"=w6343, "New_State"=10, "State Machine in"=w6338) -> ("error out"=w6342:errorcluster, "State Machine out"=w6337:refnum<class "State Machine.lvclass">)  [unwired: 7 in]
            n2672 = call-dynamic "Write State Machine.vi"("error in (no error)"=w6342, "State Machine.lvclass"=w6337, "Device in"=w6339) -> ("error out"=w6336:errorcluster, "Device out"=w6335:refnum<class "Opt_Selector.lvclass">)  [unwired: 7 in]
            n2673 = call "Write WPROT.vi"("error in (no error)"=w6336, "Opt_Selector.lvclass"=w6335, "Instrument in"=w6354) -> ("error out"=w6333:errorcluster, "Instrument out"=w6334:refnum<class "Instrument.lvclass">)  [unwired: 7 in]
            n2674 = call "Write Instrument.lvclass.vi"("error in (no error)"=w6333, "Instrument.lvclass"=w6334, "S4ACS_GUI in"=w6352) -> ("error out"=w6355:errorcluster, "S4ACS_GUI out"=w6356:refnum<class "S4GUI.lvclass">)  [unwired: 7 in]
            n2675 = call-dynamic "Write ciclos.vi"("error in (no error)"=w6355, "ciclos"=u32 0, "S4ACS_GUI in"=w6356) -> ("error out"=w6329:errorcluster, "S4ACS_GUI out"=w6330:refnum<class "S4GUI.lvclass">)  [unwired: 7 in]
          }
          frame Enabled {
            w6445 = FALSE ("Wait Until Done")
            n2676 = call <vilib>:"Application Directory.vi"() -> ("Application Directory"=w6448:path)
            n2677 = Build Path(base path=w6448, name or relative path="MsgAbortSync.vi") -> (appended path=w6449:path)
            n2678 = Open VI Reference(vi path=w6449, error in (no error)=w6443) -> (vi reference=w6447:refnum<vi>, error out=w6446:errorcluster)  [unwired: 4 in]
            n2679 = invoke class="VI" method="Run VI"(reference=w6447, error in=w6446, "Wait until done"=w6445, "Auto Dispose Ref"=w6445) -> (error out=w6442:errorcluster)  [unwired: 1 in, 4 out]
          }
        }
        n2680 = property on="#Cycles Done" class="Slide (strict)"(error in=w6323, "Scale.Maximum"=w6325, "Scale.Minimum"=w6325) -> (error out=w6326:errorcluster)  [unwired: 1 in, 1 out]
      }
      event "Pause SM": Value Change {
        n2681 = event-data() -> ()  [unwired: 1 in, 6 out]
        n2682 = disable-structure shown="Enabled" {
          disable-tunnel: w6453 -> [w6465 w6474]
          disable-tunnel: w6452 -> [w6464 w6475]
          disable-tunnel: [w6455 w6474] -> w6451
          disable-tunnel: [w6454 w6473] -> w6450
          frame Disabled {
            n2683 = disable-structure shown="Enabled" {
              disable-tunnel: w6465 -> [w6469 w6472]
              disable-tunnel: w6464 -> [w6468 w6471]
              disable-tunnel: [w6467 w6472] -> w6458
              disable-tunnel: [w6466 w6471] -> w6457
              frame Disabled {
                n2684 = call-dynamic "Write paused.vi"("error in (no error)"=w6468, "paused"=TRUE ("stopped"), "S4ACS_GUI in"=w6469) -> ("error out"=w6466:errorcluster, "S4ACS_GUI out"=w6467:refnum<class "S4GUI.lvclass">)  [unwired: 7 in]
              }
              frame Enabled {
              }
            }
            n2685 = call-dynamic "Read Obs_state.vi"("error in (no error)"=w6457, "S4ACS_GUI in"=w6458) -> ("error out"=w6461:errorcluster, "Obs_state"=w6463:u32, "S4ACS_GUI out"=w6462:refnum<class "S4GUI.lvclass">)  [unwired: 7 in]
            n2686 = call-dynamic "Write Obs_prevstate.vi"("error in (no error)"=w6461, "Obs_prevstate"=w6463, "S4ACS_GUI in"=w6462) -> ("error out"=w6459:errorcluster, "S4ACS_GUI out"=w6460:refnum<class "S4GUI.lvclass">)  [unwired: 7 in]
            n2687 = call-dynamic "Write Obs_state.vi"("error in (no error)"=w6459, "Obs_state"=u32 400, "S4ACS_GUI in"=w6460) -> ("error out"=w6454:errorcluster, "S4ACS_GUI out"=w6455:refnum<class "S4GUI.lvclass">)  [unwired: 7 in]
          }
          frame Enabled {
            w6477 = FALSE ("Wait Until Done")
            n2688 = call <vilib>:"Application Directory.vi"() -> ("Application Directory"=w6480:path)
            n2689 = Build Path(base path=w6480, name or relative path="MsgPauseSync.vi") -> (appended path=w6481:path)
            n2690 = Open VI Reference(vi path=w6481, error in (no error)=w6475) -> (vi reference=w6479:refnum<vi>, error out=w6478:errorcluster)  [unwired: 4 in]
            n2691 = invoke class="VI" method="Run VI"(reference=w6479, error in=w6478, "Wait until done"=w6477, "Auto Dispose Ref"=w6477) -> (error out=w6473:errorcluster)  [unwired: 1 in, 4 out]
          }
        }
      }
      event "Abort ch1": Value Change {
        n2692 = event-data() -> ()  [unwired: 1 in, 6 out]
        n2693 = disable-structure shown="Enabled" {
          disable-tunnel: w6485 -> [w6518 w6540]
          disable-tunnel: w6484 -> [w6516 w6533]
          disable-tunnel: [w6498 w6532] -> w6483
          disable-tunnel: [w6486 w6540] -> w6482
          frame Disabled {
            # "Para movimento \nda lamina retardadora"
            # "Restaura a última sequência de lâminas"
